vi "Procesamiento.vi"() -> ()   [LabVIEW 2014]
uses:
  <vilib>/Platform/TimedLoop/XDataNode/timing_clust.ctl
  <vilib>/Platform/TimedLoop/XDataNode/nitl_modes.ctl
  <vilib>/Platform/TimedLoop/XDataNode/wakeup.ctl
  <vilib>/FPGAPlugInAG/myRIO-1900/niLvFpga_Open_myRIO-1900.vi
  <vilib>/rvi/interface/common/dynamic/niFpgaDynamicAddResources.vi
  <vilib>/FPGAPlugInAG/Dynamic/niLvFpga_Run_Dynamic.vi
  <vilib>/rvi/interface/common/niFpgaWaitOnOcc.vi
  <vilib>/Utility/error.llb/Error Cluster From Error Code.vi
  <vilib>/rvi/errors/niLvFpgaAdjustHostInterfaceError.vi
  <vilib>/rvi/interface/nirviOpenFPGA/nirviOpenFPGA.xnode
  FPGA Bitfiles/MedidorInteligen_FPGATarget_FPGA_pD4WJt1rbbQ.lvbitx
  FPGA.vi
  <vilib>/rvi/interface/nirviMethod/nirviMethod.xnode
  <vilib>/platform/TimedLoop/XDataNode/XDataNode.xnode
  <vilib>/FPGAPlugInAG/Dynamic/niLvFpga_ConfigureFifo_Dynamic.vi
  <vilib>/rvi/errors/niLvFpgaMergeErrorWithErrorCode.vi
  <vilib>/Platform/TimedLoop/XDataNode/XDNodeRunTimeDep.lvlib
  <vilib>/FPGAPlugInAG/Dynamic/niLvFpga_StartFifo_Dynamic.vi
  <vilib>/FPGAPlugInAG/Dynamic/niLvFpga_ReadFifo_Dynamic.vi
panel:
  out "Energia Acumulada":dbl
  out "# elements in queue":i32
  out "Voltaje y Corriente 2":dbl[](graph)
  out "Cons_Cor":dbl[](array[numeric])
  out "Espectro de \npotencia":dynamicdata(graph)
  out "Nivel Componentes I":dbl[](array[numeric])
  out "Voltaje y Corriente":dynamicdata(graph)
  out "Desfasaje":dbl
  out "Potencia Reactiva":dbl
  out "Ventanas muestreo":i32=1
  out "Frecuencia \nMuestreo":dbl=6000.0
  out "Numero \nde \nmuestras":u32=1000
  out "Potencia aparente":dbl
  out "Irms":dbl format="%0.2f"
  out "Vrms":dbl format="%0.2f"
  out "Cons_Vol":dbl[](array[numeric])
  out "Potencia Activa Entregada":bool
  out "Potencia Reactiva Entregada":bool
  out "Potencia Activa":dbl format="%0.2f"
  out "THD I":dbl format="%.2p"
  out "Frequencia\nFundamental":dbl format="%.2p"
  out "THD V":dbl format="%.2p"
  out "Nivel Componentes V":dbl[](array[numeric]) format="%.2p"
  out "Tiempo de loop":u32
  out "Corriente":dbl[](array[numeric]) format="%.2f"
  out "Voltaje":dbl[](array[numeric]) format="%.2f"
  out "depth Corriente":u32
  out "depth Voltaje":u32
  # "Ventana de 12 Ciclos"
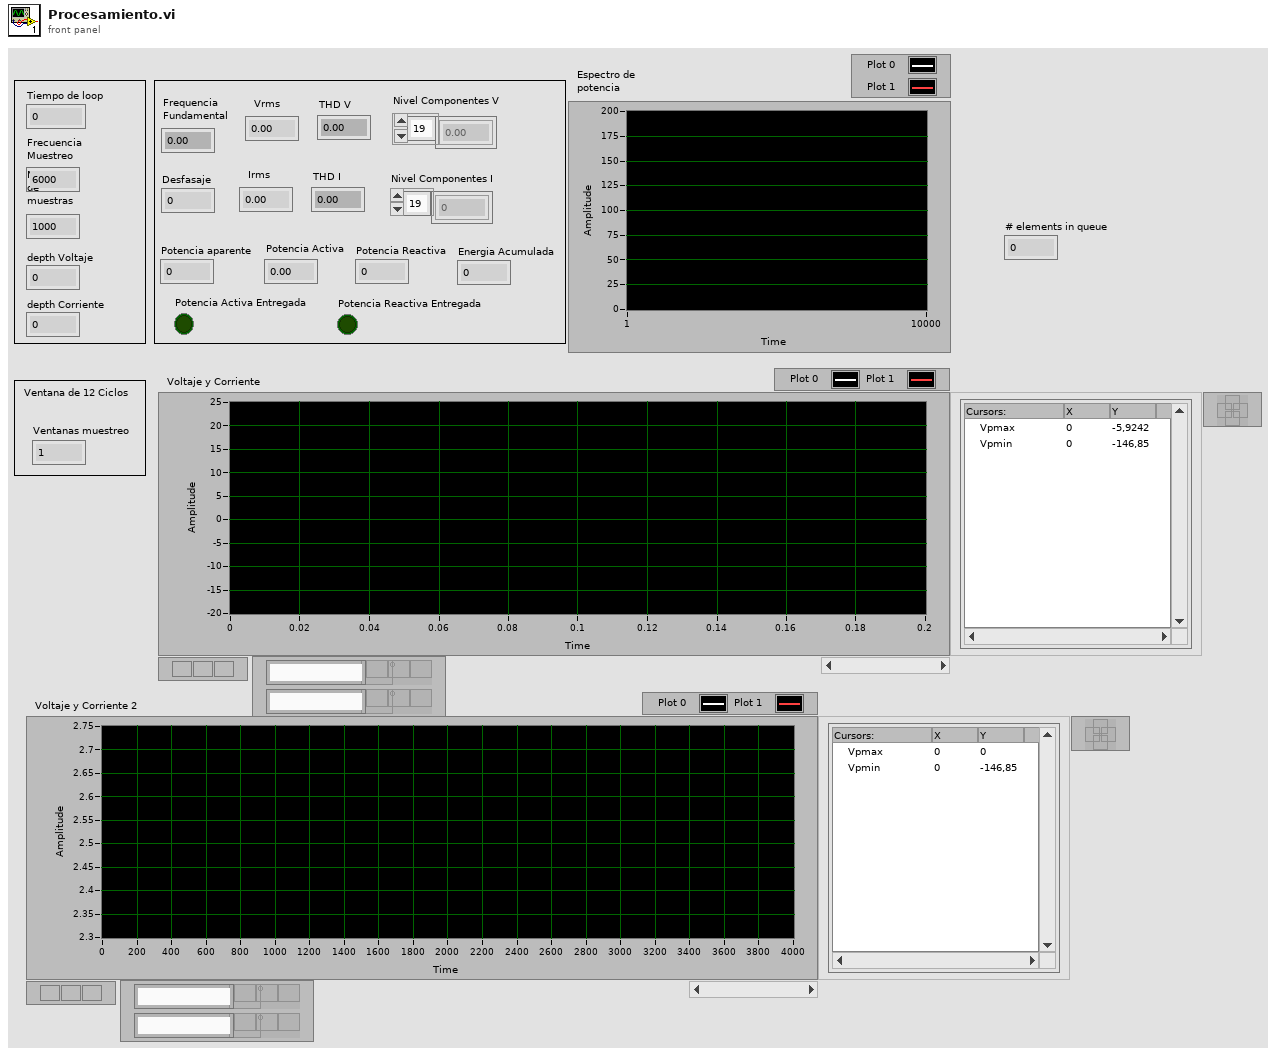
[diagram p1: front panel]
types:
  T1 = typedef "XDNodeRunTimeDep.lvlib/timing_clust.ctl" = cluster{"Expected End [f-1]":u64, "Actual End [f-1]":u64, "Finished Late? [f-1]":bool, "Expected End [i-1]":u64, "Actual End [i-1]":u64, "Finished Late? [i-1]":bool, "Expected Start [i]":u64, "Actual Start [i]":u64, "Expected Start [f]":u64, "Actual Start [f]":u64, "Source Name":string, "Structure Name":string, "Period":i64, "Deadline":i64, "Offset":i64, "Start":i64, "Priority":i32, "Timeout":i32, "Mode":T2, "Wakeup Reason":T3, "Error":errorcluster, "Source Type":string, "Secondary Source Type":string, "Global End Time":u64, "Global Start Time":u64, "Frame Duration":u64, "Iteration Duration":u64, "Assigned CPU":i32, "I/O Scan Engine Mode":u32}
  T2 = typedef "XDNodeRunTimeDep.lvlib/nitl_modes.ctl" = enum32{"No Change", "Process missed periods, maintain original phase", "Discard missed periods, maintain original phase", "Process missed periods, ignore original phase", "Discard missed periods, ignore original phase"}
  T3 = typedef "XDNodeRunTimeDep.lvlib/wakeup.ctl" = enum32{"Normal", "Aborted", "Asynchronous wakeup", "Timing source error", "Timed loop error", "Timeout"}
  T4 = cluster{"Frecuencia":dbl, "THD V":dbl, "THD I":dbl, "FDP":dbl, "Potencia Activa":dbl, "Potencia Reactiva":dbl, "Potencia Aparente":dbl, "Desfasaje (FDP)":dbl, "Desfasaje (TM)":dbl, "Flujo":dbl, "Vrms":dbl, "Irms":dbl, "Energia":dbl}
  T5 = cluster{"components level":dbl[], "Waveform":waveform(dbl), "Power Spectrum (V^2 rms)":dbl[]}
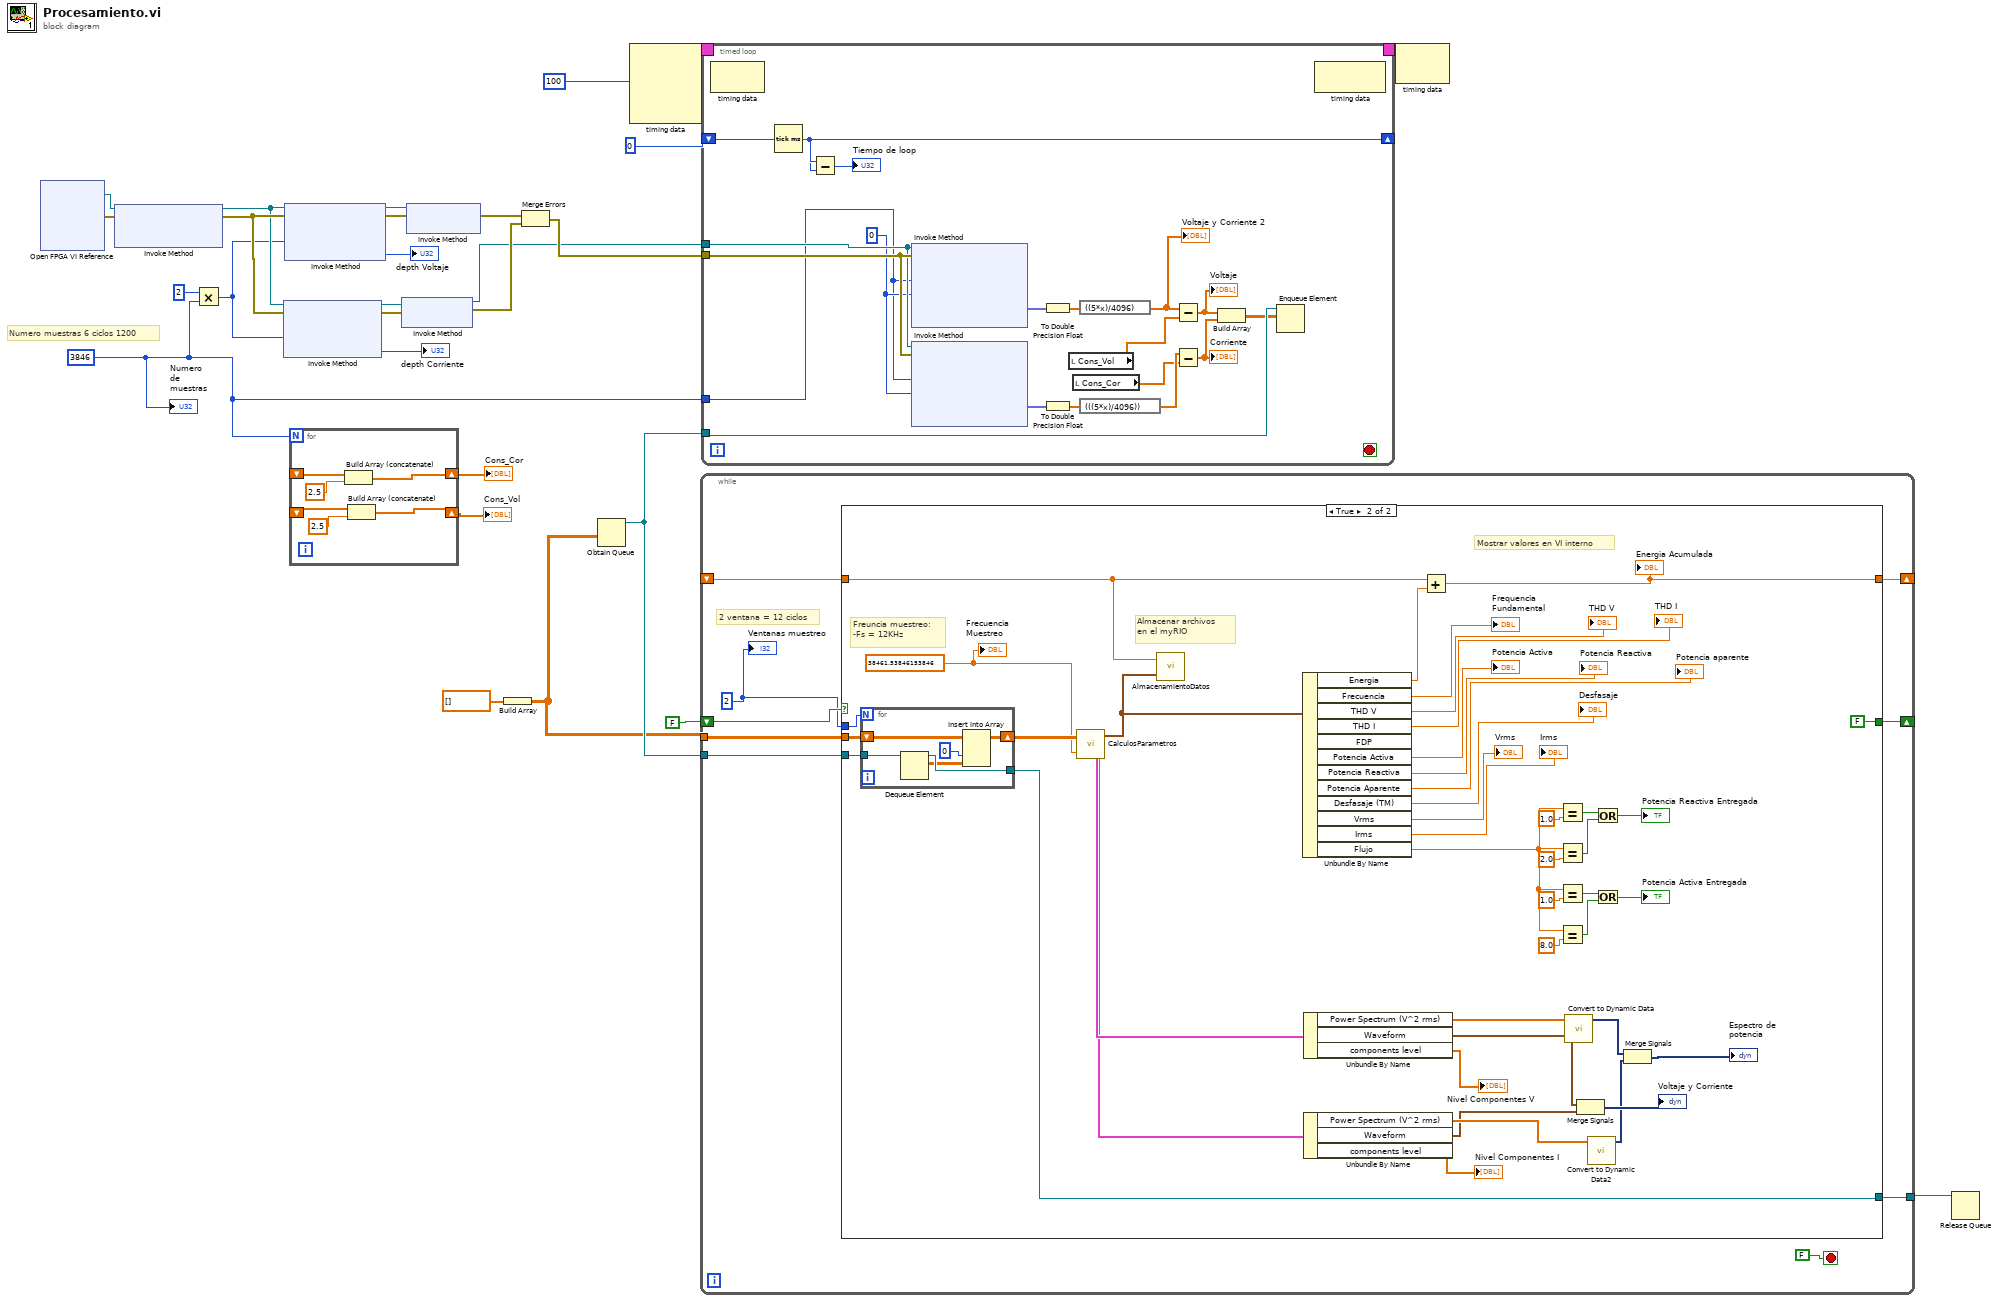
[diagram p0: block diagram]
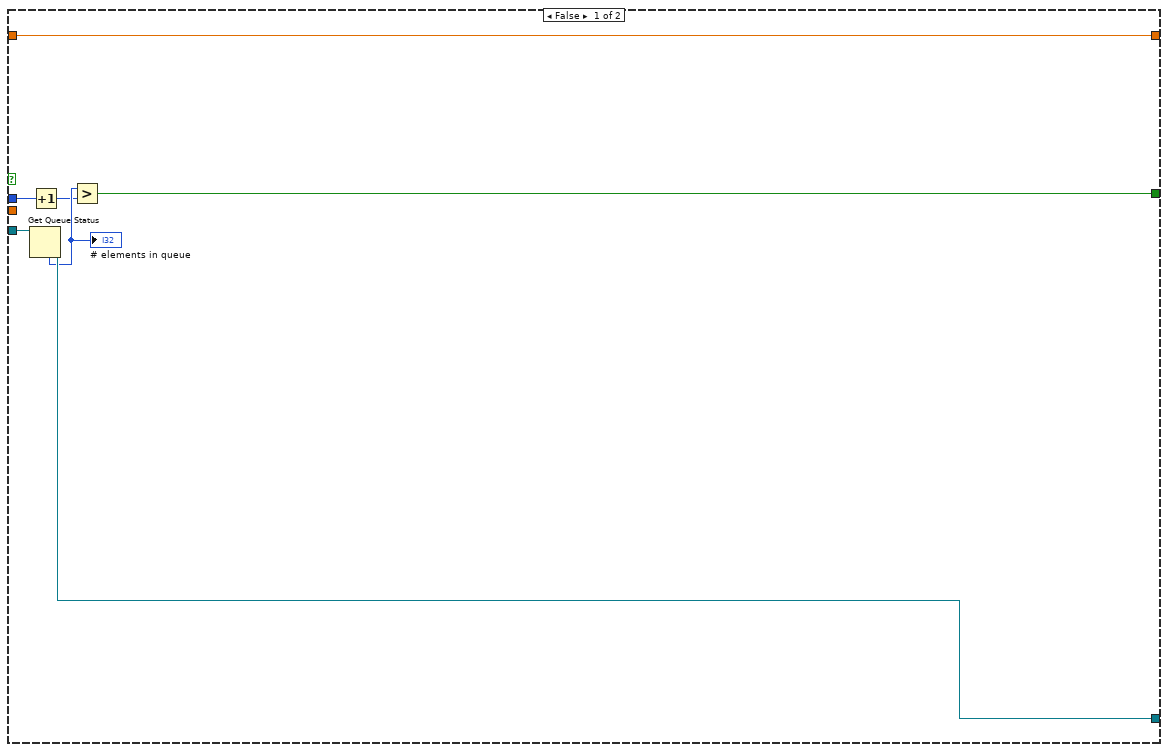
[diagram p2: hidden frame]
diagram:
  w3 = u32 3846 ("Numero de muestras")
  # "Numero muestras 6 ciclos 1200"
  n1 = xnode "Open FPGA VI Reference"() -> ("FPGA VI Reference Out"=w28:refnum<k20>, "error out"=w27:errorcluster)  [unwired: 2 in]
  n2 = xnode "Invoke Method"("FPGA VI Reference In"=w28, "error in"=w27) -> ("FPGA VI Reference Out"=w22:refnum<k20>, "error out"=w23:errorcluster)  [unwired: 1 in]
  n3 = Multiply(x=u32 2, y=w3) -> (x*y=w2:u32)
  n4 = xnode "Invoke Method"("FPGA VI Reference In"=w22, "error in"=w23, "Requested Depth"=w2) -> ("FPGA VI Reference Out"=w19:refnum<k20>, "error out"=w18:errorcluster, "Actual Depth"=→"depth Corriente":u32)
  n5 = xnode "Invoke Method"("FPGA VI Reference In"=w22, "error in"=w23, "Requested Depth"=w2) -> ("FPGA VI Reference Out"=w21:refnum<k20>, "error out"=w20:errorcluster, "Actual Depth"=→"depth Voltaje":u32)
  n6 = for {
    N: w3 -> [_]
    shift-right: [w34] -> w5
    shift-left: _ -> [w32]
    shift-right: [w29] -> w4
    shift-left: _ -> [w30]
    n7 = Build Array (concatenate)(w32, 2.5 ("element")) -> (w34:dbl[])
    n8 = Build Array (concatenate)(w30, 2.5 ("element")) -> (w29:dbl[])
  }
  "Cons_Vol" <- w4
  "Cons_Cor" <- w5
  n9 = xnode "Invoke Method"("FPGA VI Reference In"=w19, "error in"=w18) -> ("FPGA VI Reference Out"=w12:refnum<k20>, "error out"=w14:errorcluster)
  n10 = xnode "Invoke Method"("FPGA VI Reference In"=w21, "error in"=w20) -> ("error out"=w15:errorcluster)  [unwired: 1 out]
  n11 = Build Array(dbl[] []) -> (w6:dbl[][])
  n12 = Merge Errors(w15, w14) -> (w13:errorcluster)
  n13 = Obtain Queue(element data type=w6) -> (queue out=w8:refnum<queue>)  [unwired: 4 in, 2 out]
  n14 = node-c288(i64 100 ("Period")) -> (w26:T1)  [unwired: 3 in]
  n15 = while {
    shift-right: [w42] -> _
    shift-left: FALSE -> [w43]
    tunnel: w8 -> [w41]
    tunnel: [w40] -> w9
    tunnel: w6 -> [w37]
    shift-right: [w36] -> _
    shift-left: _ -> [w35]
    stop <- FALSE stop-if-true
    w38 = 2 ("Ventanas muestreo")
    # "2 ventana = 12 ciclos"
    n16 = case shown="True" w43 {
      tunnel: [w47 FALSE] -> w42
      tunnel: w41 -> [w50 w92]
      tunnel: [w49 w93] -> w40
      tunnel: w38 -> [w46 w91]
      tunnel: w37 -> [_ w89]
      tunnel: [w44 w52] -> w36
      tunnel: w35 -> [w44 w51]
      frame False {
        n17 = Get Queue Status(queue=w50) -> (queue out=w49:refnum<queue>, # elements in queue=w48:i32)  [unwired: 2 in, 6 out]
        "# elements in queue" <- w48
        n18 = Increment(x=w46) -> (x+1=w45:i32)
        n19 = Greater?(x=w48, y=w45) -> (0:w47:bool)
      }
      frame True {
        w54 = 38461.53846153846 ("Frecuencia \nMuestreo")
        # "Freuncia muestreo:\n-Fs = 12KHz"
        # "Mostrar valores en VI interno"
        # "Almacenar archivos \nen el myRIO"
        n20 = for {
          N: w91 -> [_]
          tunnel: [w99] -> w93
          tunnel: w92 -> [w98]
          shift-right: [w95] -> w87
          shift-left: w89 -> [w97]
          n21 = Dequeue Element(queue=w98) -> (queue out=w99:refnum<queue>, element=w96:dbl[][])  [unwired: 2 in, 2 out]
          n22 = Insert Into Array(array=w97, index (col)=0 ("disabled index (col)"), new element=w96) -> (w95:dbl[][])  [unwired: 1 in]
        }
        n23 = call "CalculosParametros.vi"("2D Array"=w87, "Frecuencia \nMuestreo"=w54) -> ("output cluster"=w55:T4, "Voltaje"=w86:T5, "Corriente"=w85:T5)
        n24 = call "AlmacenamientoDatos.vi"("Datos a almacenar"=w55, "Energia"=w51) -> ()  [unwired: 1 out]
        n25 = Unbundle By Name(w55) -> ("Energia"=w53:dbl, "Frecuencia"=→"Frequencia\nFundamental":dbl, "THD V"=→"THD V":dbl, "THD I"=→"THD I":dbl, "Potencia Activa"=→"Potencia Activa":dbl, "Potencia Reactiva"=→"Potencia Reactiva":dbl, "Potencia Aparente"=→"Potencia aparente":dbl, "Desfasaje (TM)"=→"Desfasaje":dbl, "Vrms"=→"Vrms":dbl, "Irms"=→"Irms":dbl, "Flujo"=w67:dbl)  [unwired: 1 out]
        n26 = Unbundle By Name(w86) -> ("Power Spectrum (V^2 rms)"=w59:dbl[], "Waveform"=w57:waveform(dbl), "components level"=→"Nivel Componentes V":dbl[])
        n27 = Unbundle By Name(w85) -> ("Power Spectrum (V^2 rms)"=w64:dbl[], "Waveform"=w56:waveform(dbl), "components level"=→"Nivel Componentes I":dbl[])
        n28 = Add(x=w51, y=w53) -> (x+y=w52:dbl)
        "Energia Acumulada" <- w52
        n29 = Equal?(x=w67, y=1.0) -> (x = y?=w73:bool)
        n30 = Equal?(x=w67, y=2.0) -> (x = y?=w71:bool)
        n31 = Equal?(x=w67, y=1.0) -> (x = y?=w70:bool)
        n32 = Equal?(x=w67, y=8.0) -> (x = y?=w69:bool)
        n33 = call "Convert to Dynamic Data"("Array"=w59) -> ("Dynamic Data Type"=w62:dynamicdata)  [unwired: 3 in]
        n34 = Merge Signals(w57, w56) -> (→"Voltaje y Corriente":dynamicdata)
        n35 = call "Convert to Dynamic Data2"("Array"=w64) -> ("Dynamic Data Type"=w60:dynamicdata)  [unwired: 3 in]
        n36 = Or(x=w73, y=w71) -> (x .or. y?=→"Potencia Reactiva Entregada":bool)
        n37 = Or(x=w70, y=w69) -> (x .or. y?=→"Potencia Activa Entregada":bool)
        n38 = Merge Signals(w62, w60) -> (→"Espectro de \npotencia":dynamicdata)
        "Frecuencia \nMuestreo" <- w54
      }
    }
    "Ventanas muestreo" <- w38
  }
  n39 = timed-loop {
    timing: w26 -> [_]
    timing-out: [_] -> w25
    tunnel: w13 -> [w118]
    tunnel: w12 -> [w117]
    shift-right: [w111] -> _
    shift-left: u32 0 ("millisecond timer value") -> [w110]
    tunnel: w8 -> [w108]
    tunnel: w3 -> [w104]
    stop <- _ stop-if-true
    w116 = 0 ("Timeout (ms)")
    n40 = node-c288() -> ()  [unwired: 1 in, 1 out]
    n41 = Tick Count (ms)() -> (millisecond timer value=w111:u32)
    n42 = Subtract(x=w111, y=w110) -> (x-y=→"Tiempo de loop":u32)
    n43 = xnode "Invoke Method"("FPGA VI Reference In"=w117, "error in"=w118, "Number of Elements"=w104, "Timeout (ms)"=w116) -> ("Data"=w115:fxp<+,16,16>[])  [unwired: 3 out]
    n44 = xnode "Invoke Method"("FPGA VI Reference In"=w117, "error in"=w118, "Number of Elements"=w104, "Timeout (ms)"=w116) -> ("Data"=w113:fxp<+,16,16>[])  [unwired: 3 out]
    n45 = To Double Precision Float(number=w115) -> (double precision float=w114:dbl[])
    n46 = To Double Precision Float(number=w113) -> (double precision float=w112:dbl[])
    n47 = local read "Cons_Vol"() -> (w102:dbl[])
    n48 = local read "Cons_Cor"() -> (w101:dbl[])
    n49 = expression code="((5*x)/4096)"(w114) -> (w100:dbl[])
    "Voltaje y Corriente 2" <- w100
    n50 = expression code="(((5*x)/4096))"(w112) -> (w107:dbl[])
    n51 = Subtract(x=w100, y=w102) -> (x-y=w103:dbl[])
    "Voltaje" <- w103
    n52 = Subtract(x=w107, y=w101) -> (x-y=w106:dbl[])
    "Corriente" <- w106
    n53 = Build Array(w103, w106) -> (w105:dbl[][])
    n54 = Enqueue Element(queue=w108, element=w105) -> ()  [unwired: 2 in, 3 out]
    n55 = node-c288() -> ()  [unwired: 1 in, 1 out]
  }
  n56 = node-c288(w25) -> ()  [unwired: 1 out]
  n57 = Release Queue(queue=w9) -> ()  [unwired: 2 in, 3 out]
  "Numero \nde \nmuestras" <- w3
